vi "Clear.vi"(3 "((Pointer)) in":refnum<class "((Pointer)).lvclass">) -> (1 "((Pointer)) out":refnum<class "((Pointer)).lvclass">)   [LabVIEW 2016, in "((Pointer)).lvclass"]
uses:
  ((Pointer)).lvclass
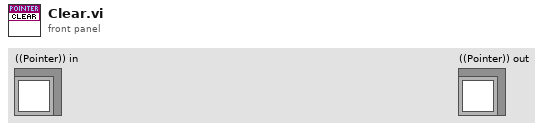
[diagram p1: front panel]
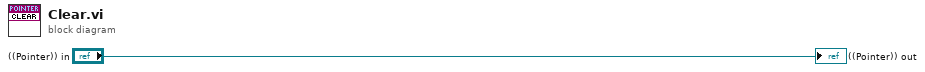
[diagram p0: block diagram]
diagram:
  "((Pointer)) out" <- "((Pointer)) in"
